vi "response.get.vi"(8 "error in (no error)":errorcluster, 9 "buf_len":i32, 10 "buf_ptr":string, 11 "handle":cluster{}) -> (0 "error out":errorcluster, 2 "buf_ptr out":string, 3 "function return":i32)   [LabVIEW 2020, in "reqwest-labview.lvlib"]
doc: "Copies a stored response body into a caller-allocated buffer and frees the handle; allocate the buffer using the response length returned by the originating request call.\n\n\n\n\n\n\nint http_read_response(unsigned long long handle,\n unsigned char *buf_ptr,\n int buf_len);"
uses:
  reqwest-labview.lvlib
  http_rs_labview.dll
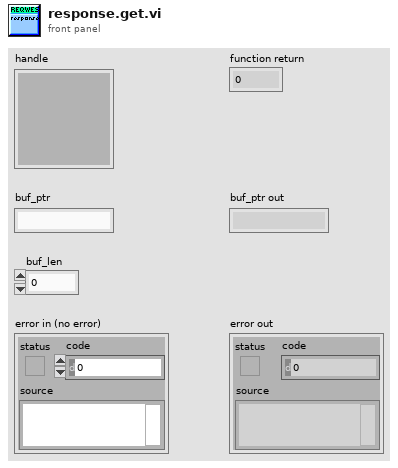
[diagram p1: front panel]
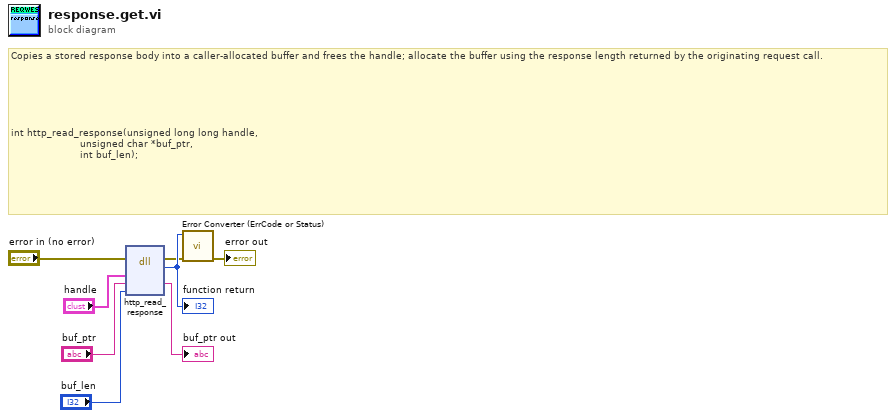
[diagram p0: block diagram]
diagram:
  # "Copies a stored response body into a caller-allocated buffer and frees the handle; allocate the buffer using the response length returned by the originating request call.\n\n\n\n\n\n\nint http_read_response(unsigned long long handle,\n                       unsigned char *buf_ptr,\n                       int buf_len);"
  n1 = dll-call lib="C:/code/reqwest-labview/lv-src/shared-library/http_rs_labview.*" fn="http_read_response"(error in="error in (no error)", "handle"="handle", "buf_ptr"="buf_ptr", "buf_len"="buf_len") -> (error out=w2:errorcluster, w8:i32, "buf_ptr"=→"buf_ptr out":string)  [unwired: 4 in, 1 out]
  "function return" <- w8
  n2 = call "Error Converter (ErrCode or Status).vi"("error in (no error)"=w2, "error code"=w8) -> ("error out"=→"error out":errorcluster)  [unwired: 9 in]
